vi "LVClass_CorrectionDataManager GetActuatorPrefs.vi"(0 "CorrectionDataManager in":refnum<class "CorrectionDataManager.lvclass">, 5 "N° actuator":i32, 11 "error in (no error)":errorcluster) -> (4 "CorrectionDataManager out":refnum<class "CorrectionDataManager.lvclass">, 6 "Actuator state":T1, 15 "error out":errorcluster)   [LabVIEW 2020, in "CorrectionDataManager.lvclass"]
doc: "Preferences getter for one wavefront corrector actuator.\n\n<B>corrdata_managerIn</B> : CorrDataManager object\n<B>corrdata_managerOut</B> : CorrDataManager object\n<B>actuator_index</B> : Index of the actuator.\n<B>min</B> : WavefrontCorrector actuator preferences : lowest command value.\n<B>max</B> : WavefrontCorrector actuator preferences : highest command value.\n<B>validity</B> : WavefrontCorrector actuator preferences : status.\n<B>fixed_value</B> : WavefrontCorrector actuator preferences : fixed positions."
uses:
  CorrectionDataManager.lvclass
  Controls/Wavefront Corrector states - ONE.ctl
  CorrectionDataManager.lvclass/CorrectionDataManager.ctl
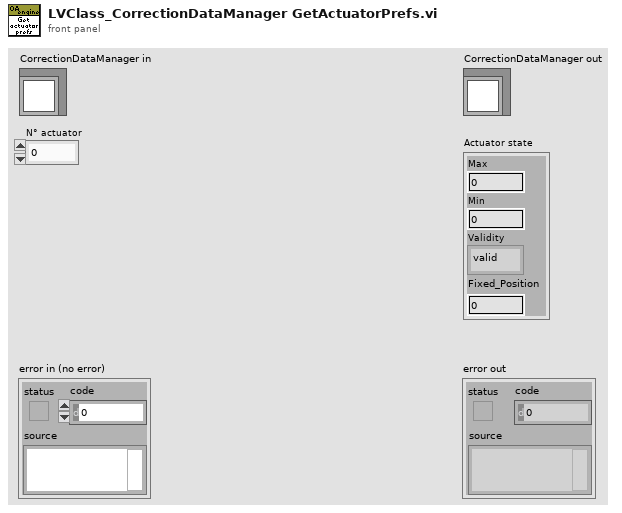
[diagram p1: front panel]
types:
  T1 = typedef "Wavefront Corrector states - ONE.ctl" = cluster{"Max":sgl, "Min":sgl, "Validity":enum16{"valid", "fixed", "invalid"}, "Fixed_Position":sgl}
  T2 = typedef "ClassID.ctl" = i64
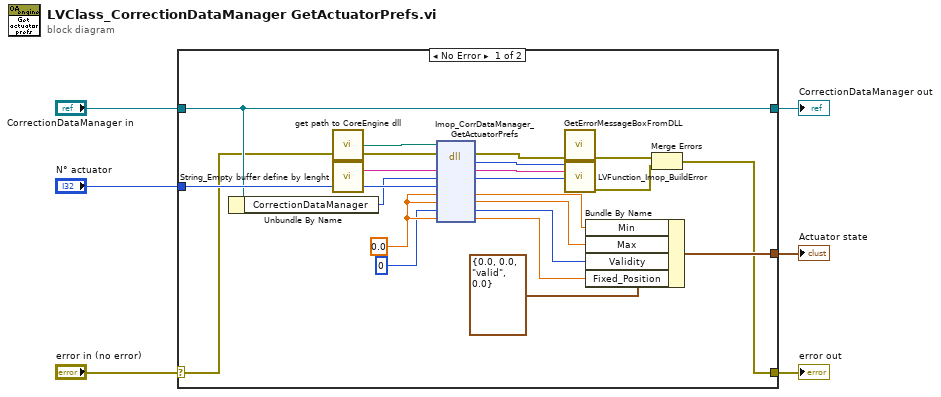
[diagram p0: block diagram]
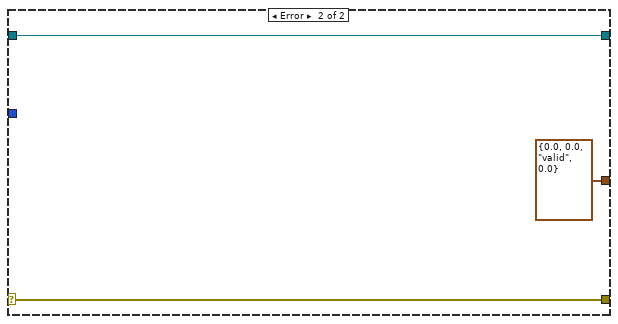
[diagram p2: hidden frame]
diagram:
  n1 = case shown="No Error" "error in (no error)" {
    selector: "error in (no error)" -> [w9 w30]
    tunnel: [w8 w30] -> w5
    tunnel: [w19 w29] -> w3
    tunnel: "CorrectionDataManager in" -> [w19 w29]
    tunnel: "N° actuator" -> [w20 _]
    tunnel: [w10 T1 {"Max"=0.0, "Min"=0.0, "Validity"=enum."valid", "Fixed_Position"=0.0} ("Actuator state")] -> w1
    frame No Error {
      w17 = 0.0
      n2 = Unbundle By Name(w19) -> ("CorrectionDataManager"=w18:T2)
      n3 = call "get path to CoreEngine dll.vi"() -> ("path to wavekit library"=w25:path)  [unwired: 14 in, 1 out]
      n4 = call "String_Empty buffer define by lenght.vi"() -> ("Empty buffer"=w24:string)  [unwired: 1 in]
      n5 = dll-call lib="D:/FLE/0.Code/CoreEngine4_Suite/LV2011_interface/DLLs/c_interface_vc100.dll" fn="Imop_CorrDataManager_GetActuatorPrefs"(path in=w25, error in=w9, "Message"=w24, "CorrectionDataManager"=w18, "Actuator index"=w20, "Min"=w17, "Max"=w17, "Validity"=0, "Fixed position"=w17) -> (error out=w23:errorcluster, "return type"=w22:i32, "Message"=w21:string, "CorrectionDataManager"=w7:i64, "Min"=w14:sgl, "Max"=w13:sgl, "Validity"=w12:i32, "Fixed position"=w11:sgl)  [unwired: 2 in, 1 out]
      n6 = call "GetErrorMessageBoxFromDLL.vi"("error IN"=w23) -> ("error OUT"=w27:errorcluster)  [unwired: 10 in]
      n7 = call "LVFunction_Imop_BuildError.vi"("code"=w22, "String to Prepend to source (\"\")"=w21, "Adresse"=w7) -> ("error out"=w26:errorcluster)  [unwired: 12 in]
      n8 = Bundle By Name(cluster=T1 {"Max"=0.0, "Min"=0.0, "Validity"=enum."valid", "Fixed_Position"=0.0} ("Actuator state"), "Min"=w14, "Max"=w13, "Validity"=w12, "Fixed_Position"=w11) -> (w10:T1)
      n9 = Merge Errors(w27, w26) -> (w8:errorcluster)
    }
    frame Error {
    }
  }
  "error out" <- w5
  "CorrectionDataManager out" <- w3
  "Actuator state" <- w1
